vi "Enter set temperature in Celcius.vi"(8 "error in (no error)":errorcluster, 10 "Temperature (C)":u16, 11 "VISA resource name":refnum<visa-resource-name>) -> (0 "error out":errorcluster, 3 "VISA resource name out":refnum<visa-resource-name>)   [LabVIEW 2018]
panel:
  out "resulting string":string
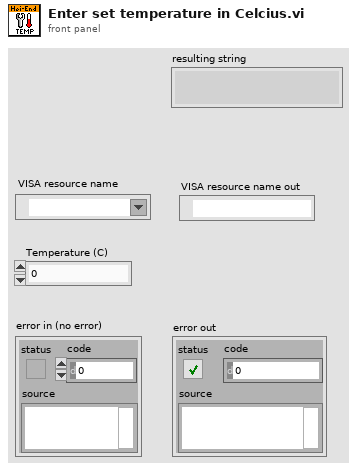
[diagram p1: front panel]
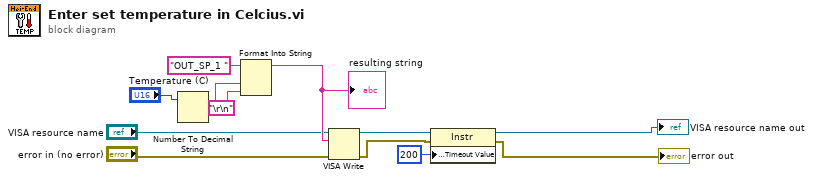
[diagram p0: block diagram]
diagram:
  n1 = Number To Decimal String(number="Temperature (C)") -> (decimal integer string=w1:string)  [unwired: 1 in]
  n2 = Format Into String(initial string="OUT_SP_1 ", w1, "\r\n") -> (resulting string=w11:string)  [unwired: 2 in, 1 out]
  "resulting string" <- w11
  n3 = VISA Write(VISA resource name="VISA resource name", write buffer=w11, error in (no error)="error in (no error)") -> (VISA resource name out=w7:refnum<visa-resource-name>, error out=w6:errorcluster)  [unwired: 1 out]
  n4 = property class="Instr"(reference=w7, error in=w6, "General Settings:Timeout Value"=u32 200) -> (reference out=→"VISA resource name out":refnum<visa-resource-name>, error out=→"error out":errorcluster)
